vi "ChannelSettings.vi"() -> ()   [LabVIEW 2018]
panel:
  in  "Enable all":bool
  in  "RangeAll":dbl(ring) items=["0.2 Vpp"=2.0, "0.4 Vpp"=4.0, "0.8 Vpp"=8.0, "2 Vpp"=20.0, "4 Vpp"=40.0, "8 Vpp"=80.0, "20 Vpp"=200.0, "40 Vpp"=400.0, "80 Vpp"=800.0]
  in  "Apply all":bool
  in  "Channel range":T1 {"RangeC16" items=["0.2 Vpp"=2.0, "0.4 Vpp"=4.0, "0.8 Vpp"=8.0, "2 Vpp"=20.0, "4 Vpp"=40.0, "8 Vpp"=80.0, "20 Vpp"=200.0, "40 Vpp"=400.0, "80 Vpp"=800.0]; "RangeC15" items=["0.2 Vpp"=2.0, "0.4 Vpp"=4.0, "0.8 Vpp"=8.0, "2 Vpp"=20.0, "4 Vpp"=40.0, "8 Vpp"=80.0, "20 Vpp"=200.0, "40 Vpp"=400.0, "80 Vpp"=800.0]; "RangeC14" items=["0.2 Vpp"=2.0, "0.4 Vpp"=4.0, "0.8 Vpp"=8.0, "2 Vpp"=20.0, "4 Vpp"=40.0, "8 Vpp"=80.0, "20 Vpp"=200.0, "40 Vpp"=400.0, "80 Vpp"=800.0]; "RangeC13" items=["0.2 Vpp"=2.0, "0.4 Vpp"=4.0, "0.8 Vpp"=8.0, "2 Vpp"=20.0, "4 Vpp"=40.0, "8 Vpp"=80.0, "20 Vpp"=200.0, "40 Vpp"=400.0, "80 Vpp"=800.0]; "RangeC12" items=["0.2 Vpp"=2.0, "0.4 Vpp"=4.0, "0.8 Vpp"=8.0, "2 Vpp"=20.0, "4 Vpp"=40.0, "8 Vpp"=80.0, "20 Vpp"=200.0, "40 Vpp"=400.0, "80 Vpp"=800.0]; "RangeC11" items=["0.2 Vpp"=2.0, "0.4 Vpp"=4.0, "0.8 Vpp"=8.0, "2 Vpp"=20.0, "4 Vpp"=40.0, "8 Vpp"=80.0, "20 Vpp"=200.0, "40 Vpp"=400.0, "80 Vpp"=800.0]; "RangeC10" items=["0.2 Vpp"=2.0, "0.4 Vpp"=4.0, "0.8 Vpp"=8.0, "2 Vpp"=20.0, "4 Vpp"=40.0, "8 Vpp"=80.0, "20 Vpp"=200.0, "40 Vpp"=400.0, "80 Vpp"=800.0]; "RangeC9" items=["0.2 Vpp"=2.0, "0.4 Vpp"=4.0, "0.8 Vpp"=8.0, "2 Vpp"=20.0, "4 Vpp"=40.0, "8 Vpp"=80.0, "20 Vpp"=200.0, "40 Vpp"=400.0, "80 Vpp"=800.0]; "RangeC8" items=["0.2 Vpp"=2.0, "0.4 Vpp"=4.0, "0.8 Vpp"=8.0, "2 Vpp"=20.0, "4 Vpp"=40.0, "8 Vpp"=80.0, "20 Vpp"=200.0, "40 Vpp"=400.0, "80 Vpp"=800.0]; "RangeC7" items=["0.2 Vpp"=2.0, "0.4 Vpp"=4.0, "0.8 Vpp"=8.0, "2 Vpp"=20.0, "4 Vpp"=40.0, "8 Vpp"=80.0, "20 Vpp"=200.0, "40 Vpp"=400.0, "80 Vpp"=800.0]; "RangeC6" items=["0.2 Vpp"=2.0, "0.4 Vpp"=4.0, "0.8 Vpp"=8.0, "2 Vpp"=20.0, "4 Vpp"=40.0, "8 Vpp"=80.0, "20 Vpp"=200.0, "40 Vpp"=400.0, "80 Vpp"=800.0]; "RangeC5" items=["0.2 Vpp"=2.0, "0.4 Vpp"=4.0, "0.8 Vpp"=8.0, "2 Vpp"=20.0, "4 Vpp"=40.0, "8 Vpp"=80.0, "20 Vpp"=200.0, "40 Vpp"=400.0, "80 Vpp"=800.0]; "RangeC4" items=["0.2 Vpp"=2.0, "0.4 Vpp"=4.0, "0.8 Vpp"=8.0, "2 Vpp"=20.0, "4 Vpp"=40.0, "8 Vpp"=80.0, "20 Vpp"=200.0, "40 Vpp"=400.0, "80 Vpp"=800.0]; "RangeC3" items=["0.2 Vpp"=2.0, "0.4 Vpp"=4.0, "0.8 Vpp"=8.0, "2 Vpp"=20.0, "4 Vpp"=40.0, "8 Vpp"=80.0, "20 Vpp"=200.0, "40 Vpp"=400.0, "80 Vpp"=800.0]; "RangeC2" items=["0.2 Vpp"=2.0, "0.4 Vpp"=4.0, "0.8 Vpp"=8.0, "2 Vpp"=20.0, "4 Vpp"=40.0, "8 Vpp"=80.0, "20 Vpp"=200.0, "40 Vpp"=400.0, "80 Vpp"=800.0]; "RangeC1" items=["0.2 Vpp"=2.0, "0.4 Vpp"=4.0, "0.8 Vpp"=8.0, "2 Vpp"=20.0, "4 Vpp"=40.0, "8 Vpp"=80.0, "20 Vpp"=200.0, "40 Vpp"=400.0, "80 Vpp"=800.0]}
  in  "Trigger?":bool[](array[boolean])
  in  "Enable?":bool[](array[boolean])
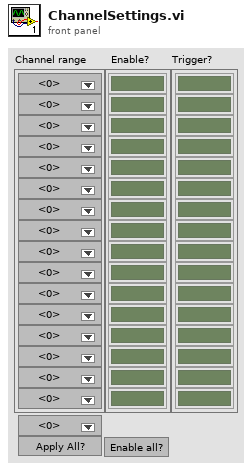
[diagram p1: front panel]
types:
  T1 = cluster{"RangeC1":dbl, "RangeC2":dbl, "RangeC3":dbl, "RangeC4":dbl, "RangeC5":dbl, "RangeC6":dbl, "RangeC7":dbl, "RangeC8":dbl, "RangeC9":dbl, "RangeC10":dbl, "RangeC11":dbl, "RangeC12":dbl, "RangeC13":dbl, "RangeC14":dbl, "RangeC15":dbl, "RangeC16":dbl}
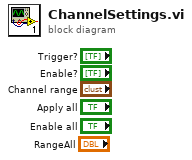
[diagram p0: block diagram]
diagram:
